vi "IZDyPos.vi"(0 "PRIORLib.IZIn":refnum<k7>, 1 "PRIORLib.IScanIn":refnum<k7>) -> (2 "PRIORLib.IZOut":refnum<k7>, 3 "PRIORLib.IScanOut":refnum<k7>, 4 "ZPos":dbl)   [LabVIEW 2011]
uses:
  Globals.vi
panel:
  out "IScanError":errorcluster
  out "IZError":errorcluster
  out "Return":u32
  out "Moving":bool
  # "This SubVi gets the Z axis position every 100 ms. while\nthe axis is moving, then returns the final Z axis location\nafter the stage stops."
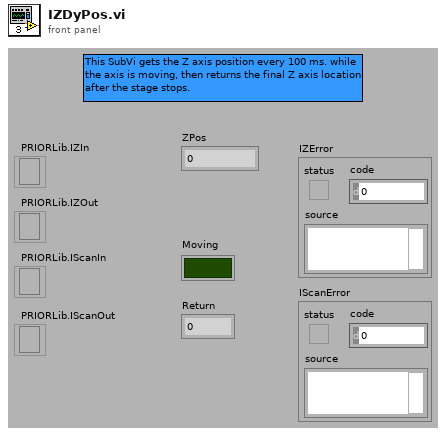
[diagram p1: front panel]
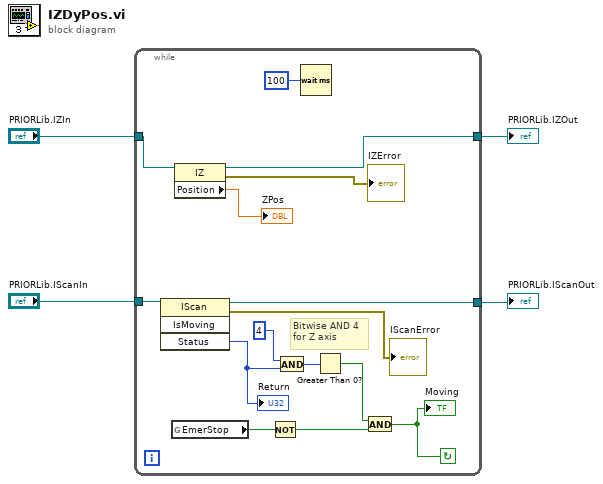
[diagram p0: block diagram]
diagram:
  n1 = while {
    tunnel: "PRIORLib.IZIn" -> [w19]
    tunnel: [w18] -> w3
    tunnel: "PRIORLib.IScanIn" -> [w16]
    tunnel: [w15] -> w1
    stop <- w6 continue-if-true
    # "Bitwise AND 4\nfor Z axis"
    n2 = invoke class="IScan" method="IsMoving"(reference=w16) -> (reference out=w15:refnum<k7>, error out=→"IScanError":errorcluster, "Status"=w5:i32)  [unwired: 3 in, 1 out]
    "Return" <- w5
    n3 = global read "Globals.vi" "EmerStop"() -> (w9:bool)
    n4 = property class="IZ"(reference=w19) -> (reference out=w18:refnum<k7>, error out=→"IZError":errorcluster, "Position"=→"ZPos":dbl)  [unwired: 1 in]
    n5 = Not(x=w9) -> (.not. x?=w7:bool)
    n6 = And(x=4, y=w5) -> (x .and. y?=w10:i32)
    n7 = Wait (ms)(milliseconds to wait=u32 100) -> ()  [unwired: 1 out]
    n8 = Greater Than 0?(x=w10) -> (x > 0?=w8:bool)
    n9 = And(x=w8, y=w7) -> (x .and. y?=w6:bool)
    "Moving" <- w6
  }
  "PRIORLib.IZOut" <- w3
  "PRIORLib.IScanOut" <- w1
